vi "Set_MG3700A_Mode_user.vi"(6 "RF output Mode (ON)":T2, 7 "Modulation Mode (ON)":T2, 8 "Error in (no error)":errorcluster, 9 "Units (dBm)":T1, 10 "N type Output Level Value (0.00)":dbl format="%.2f", 11 "VISA In":refnum<visa-resource-name>) -> (0 "Error out":errorcluster, 2 "Output Level Value out":dbl format="%.2f", 3 "VISA Out":refnum<visa-resource-name>, 4 "RF output Mode out":T2, 5 "Modulation Mode out":T2)   [LabVIEW 2015]
uses:
  MG3700A/Controls/On_Off.ctl
  MG3700A/Controls/DBM_DBU.ctl
panel:
  out "Error code":i32
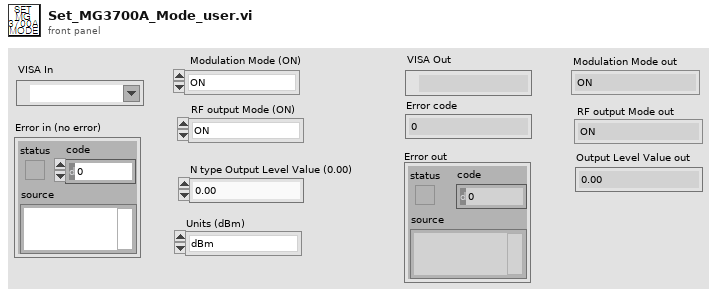
[diagram p1: front panel]
types:
  T1 = typedef "DBM_DBU.ctl" = enum16{"dBm", "dBu"}
  T2 = typedef "On_Off.ctl" = enum16{"ON", "OFF"}
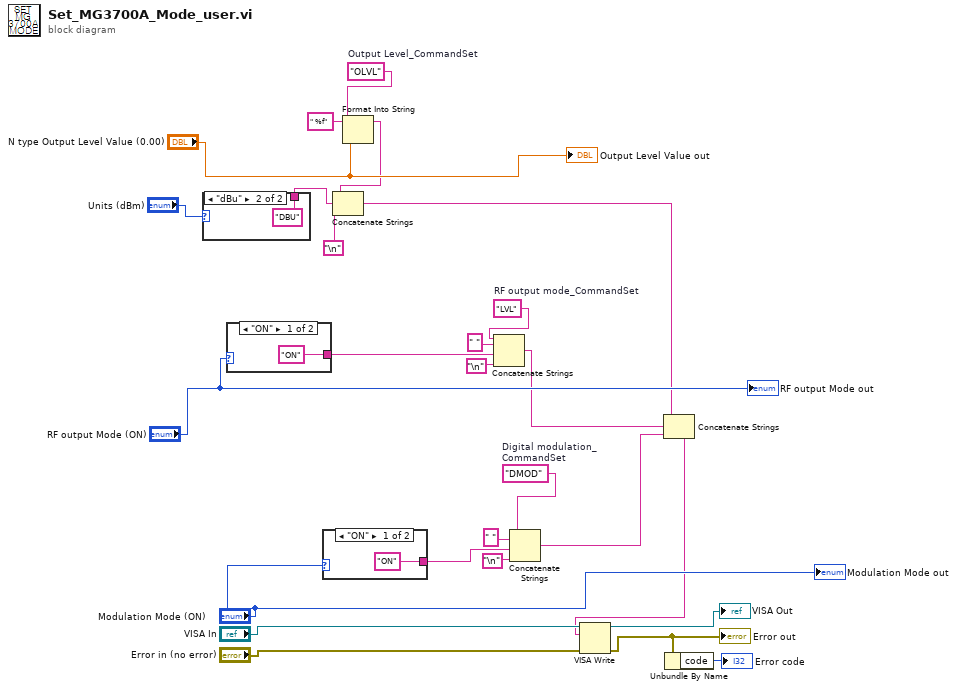
[diagram p0: block diagram]
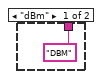
[diagram p2: hidden frame]
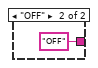
[diagram p3: hidden frame]
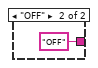
[diagram p4: hidden frame]
diagram:
  w6 = "OLVL"  # Output Level_CommandSet
  w11 = "LVL"  # RF output mode_CommandSet
  w21 = "DMOD"  # Digital modulation_CommandSet
  n1 = case shown="\"dBu\"" "Units (dBm)" {
    tunnel: ["DBM" "DBU"] -> w4
    frame "dBm" {
    }
    frame "dBu" {
    }
  }
  n2 = case shown="\"ON\"" "RF output Mode (ON)" {
    tunnel: ["ON" "OFF"] -> w12
    frame "ON" {
    }
    frame "OFF" {
    }
  }
  n3 = case shown="\"ON\"" "Modulation Mode (ON)" {
    tunnel: ["ON" "OFF"] -> w24
    frame "ON" {
    }
    frame "OFF" {
    }
  }
  n4 = Format Into String(format string=" %f" ("Format String"), initial string=w6, "N type Output Level Value (0.00)") -> (resulting string=w3:string)  [unwired: 1 in, 1 out]
  n5 = Concatenate Strings(w3, w4, "\n") -> (w1:string)
  n6 = Concatenate Strings(w11, " " ("Substring"), w12, "\n") -> (w9:string)
  n7 = Concatenate Strings(w21, " " ("Substring"), w24, "\n") -> (w16:string)
  n8 = Concatenate Strings(w1, w9, w16) -> (w15:string)
  n9 = VISA Write(VISA resource name="VISA In", write buffer=w15, error in (no error)="Error in (no error)") -> (VISA resource name out=→"VISA Out":refnum<visa-resource-name>, error out=w18:errorcluster)  [unwired: 1 out]
  "Error out" <- w18
  n10 = Unbundle By Name(w18) -> ("code"=→"Error code":i32)
  "Modulation Mode out" <- "Modulation Mode (ON)"
  "RF output Mode out" <- "RF output Mode (ON)"
  "Output Level Value out" <- "N type Output Level Value (0.00)"
